vi "test Message - Update.vi"(8 "error in (no error)":errorcluster, 11 "TestCase in":refnum<class "Test_Queue.lvclass">) -> (0 "error out":errorcluster, 3 "TestCase out":refnum<class "Test_Queue.lvclass">)   [LabVIEW 2015, in "Test_Queue.lvclass"]
uses:
  Test_Queue.lvclass
  Global Parameters.vi
  Core/Session/Session.lvclass
  Queue/NI_Azure_Queue.lvlib
  _shared/_Unit Tests Shared.lvlib
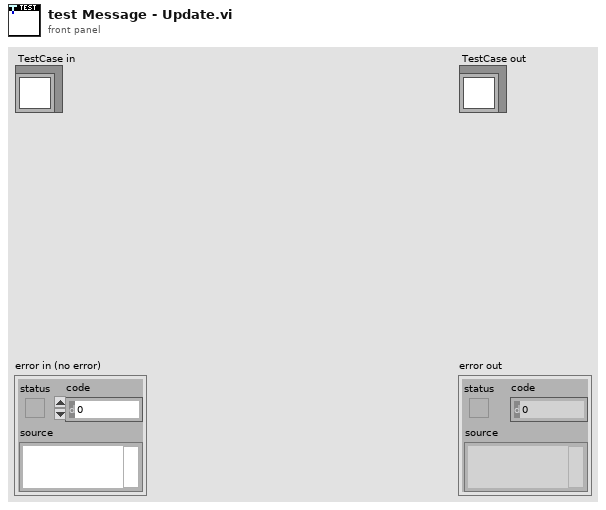
[diagram p1: front panel]
types:
  T1 = typedef "NI_Azure_Core.lvlib/Azure Credentials.ctl" = cluster{"Storage Account Name":string, "Access Key":string}
  T2 = typedef "NI_Azure_Queue.lvlib/Message.ctl" = cluster{"Message ID":string, "Insertion Time":string, "Expiration Time":string, "Pop Receipt":string, "Time Next Visible":string, "Dequeue Count":i32, "Message Text":string}
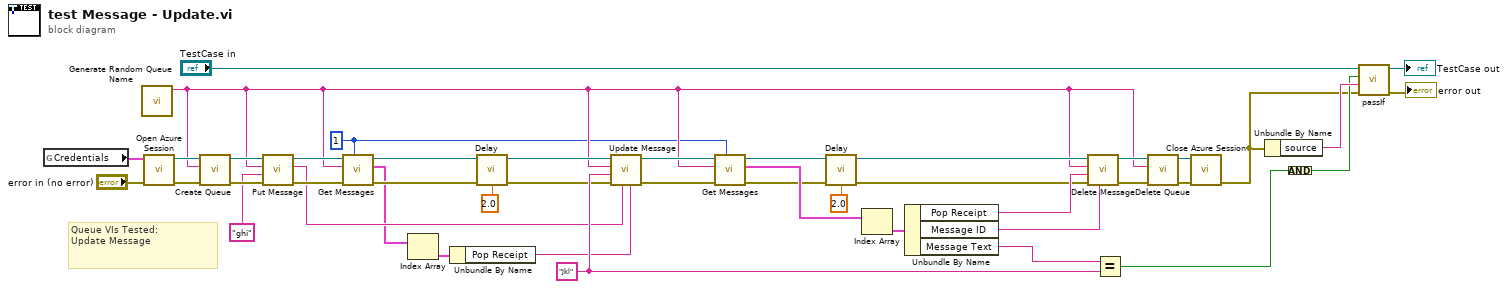
[diagram p0: block diagram]
diagram:
  w1 = u32 1 ("Visibility timeout (30 seconds)")
  w23 = "jkl"
  # "Queue VIs Tested:\nUpdate Message"
  n1 = global read "Global Parameters.vi" "Credentials"() -> (w36:T1)
  n2 = call "Generate Random Queue Name.vi"() -> ("Random Queue Name"=w5:string)  [unwired: 11 in]
  n3 = call "Open Azure Session.vi"("error in (no error)"="error in (no error)", "Credentials"=w36) -> ("error out"=w37:errorcluster, "Azure Session"=w32:refnum<class "Session.lvclass">)  [unwired: 8 in]
  n4 = call "Create Queue.vi"("error in (no error)"=w37, "Queue"=w5, "Azure Session in"=w32) -> ("error out"=w33:errorcluster, "Azure Session out"=w28:refnum<class "Session.lvclass">)  [unwired: 7 in]
  n5 = call "Put Message.vi"("error in (no error)"=w33, "Message"="ghi", "Queue"=w5, "Azure Session in"=w28) -> ("error out"=w29:errorcluster, "Message ID"=w20:string, "Azure Session out"=w17:refnum<class "Session.lvclass">)  [unwired: 5 in]
  n6 = call "Get Messages.vi"("Visibility timeout (30 seconds)"=w1, "error in (no error)"=w29, "Queue"=w5, "Azure Session in"=w17) -> ("error out"=w18:errorcluster, "Messages"=w15:T2[], "Azure Session out"=w16:refnum<class "Session.lvclass">)  [unwired: 5 in]
  n7 = Index Array(array=w15) -> (element=w14:T2)  [unwired: 1 in]
  n8 = Unbundle By Name(w14) -> ("Pop Receipt"=w13:string)
  n9 = call "Delay.vi"("error in"=w18, "delay (1 sec)"=2.0) -> ("error out"=w10:errorcluster)  [unwired: 13 in]
  n10 = call "Update Message.vi"("Pop Receipt"=w13, "Message ID"=w20, "error in (no error)"=w10, "Message"=w23, "Queue"=w5, "Azure Session in"=w16) -> ("error out"=w26:errorcluster, "Azure Session out"=w25:refnum<class "Session.lvclass">)  [unwired: 4 in]
  n11 = call "Get Messages.vi"("Visibility timeout (30 seconds)"=w1, "error in (no error)"=w26, "Queue"=w5, "Azure Session in"=w25) -> ("error out"=w3:errorcluster, "Messages"=w7:T2[], "Azure Session out"=w6:refnum<class "Session.lvclass">)  [unwired: 5 in]
  n12 = call "Delay.vi"("error in"=w3, "delay (1 sec)"=2.0) -> ("error out"=w2:errorcluster)  [unwired: 13 in]
  n13 = Index Array(array=w7) -> (element=w19:T2)  [unwired: 1 in]
  n14 = Unbundle By Name(w19) -> ("Pop Receipt"=w12:string, "Message ID"=w11:string, "Message Text"=w24:string)
  n15 = call "Delete Message.vi"("Message ID"=w11, "error in (no error)"=w2, "Pop Receipt"=w12, "Queue"=w5, "Azure Session in"=w6) -> ("error out"=w8:errorcluster, "Azure Session out"=w21:refnum<class "Session.lvclass">)  [unwired: 5 in]
  n16 = Equal?(x=w24, y=w23) -> (x = y?=w22:bool)
  n17 = call "Delete Queue.vi"("error in (no error)"=w8, "Queue"=w5, "Azure Session in"=w21) -> ("error out"=w31:errorcluster, "Azure Session out"=w30:refnum<class "Session.lvclass">)  [unwired: 7 in]
  n18 = call "Close Azure Session.vi"("error in (no error)"=w31, "Azure Session"=w30) -> ("error out"=w34:errorcluster)  [unwired: 9 in]
  n19 = Unbundle By Name(w34) -> ("source"=w39:string)
  n20 = Compound Arithmetic op=AND(w22) -> (w35:bool)
  n21 = call-dynamic "passIf.vi"("error in (no error)"=w34, "message (\"\")"=w39, "pass"=w35, "TestCase in"="TestCase in") -> ("error out"=→"error out":errorcluster, "TestCase out"=→"TestCase out":refnum<class "Test_Queue.lvclass">)  [unwired: 6 in]
